vi "Filter.vi"(8 "error in (no error)":errorcluster, 10 "Input":sgl[][](array[numeric]), 11 "Std. Deviation in":refnum<class "Std. Deviation.lvclass">) -> (0 "error out":errorcluster, 2 "Output":sgl[][](array[numeric]), 3 "Std. Deviation out":refnum<class "Std. Deviation.lvclass">)   [LabVIEW 2015, in "Std. Deviation.lvclass"]
uses:
  Std. Deviation.lvclass
  Std. Deviation.lvclass/Std. Deviation.ctl
  Filter.lvclass
  <vilib>/Analysis/NI_AALBase.lvlib
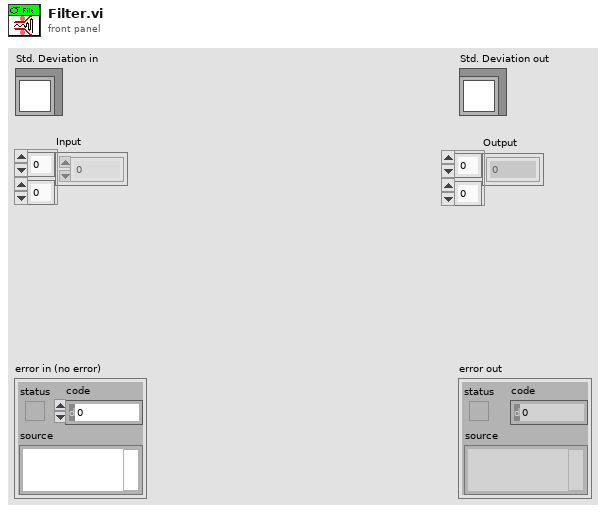
[diagram p1: front panel]
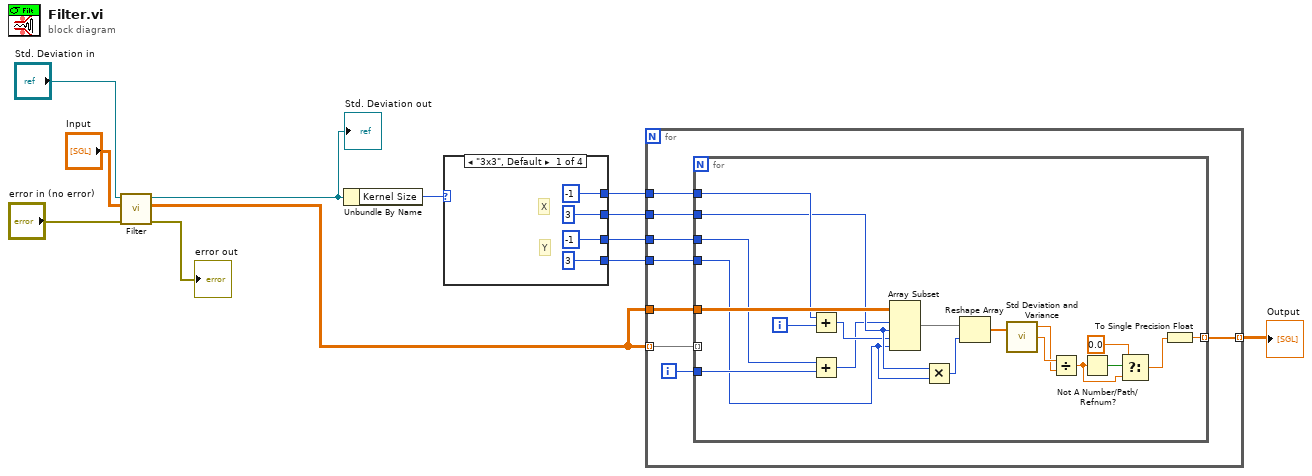
[diagram p0: block diagram]
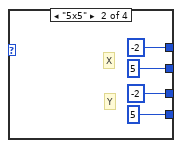
[diagram p2: hidden frame]
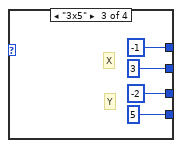
[diagram p3: hidden frame]
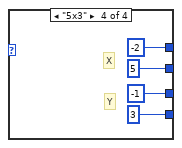
[diagram p4: hidden frame]
diagram:
  n1 = call-parent "Filter.vi"("error in (no error)"="error in (no error)", "Input"="Input", "Filter in"="Std. Deviation in") -> ("error out"=→"error out":errorcluster, "Output"=w7:sgl[][], "Filter out"=w1:refnum<class "Std. Deviation.lvclass">)  [unwired: 6 in]
  "Std. Deviation out" <- w1
  n2 = Unbundle By Name(w1) -> ("Kernel Size"=w8:enum16{"3x3", "5x5", "3x5", "5x3"})
  n3 = case shown="\"3x3\", Default" w8 {
    tunnel: [-1 -2 -1 -2] -> w6
    tunnel: [3 5 3 5] -> w5
    tunnel: [-1 -2 -2 -1] -> w4
    tunnel: [3 5 5 3] -> w3
    frame "3x3", Default {
      # "Y"
      # "X"
    }
    frame "5x5" {
      # "Y"
      # "X"
    }
    frame "3x5" {
      # "Y"
      # "X"
    }
    frame "5x3" {
      # "Y"
      # "X"
    }
  }
  n4 = for {
    tunnel: w7 -> [w36] mode=indexing
    tunnel: w7 -> [w35]
    tunnel: w6 -> [w34]
    tunnel: w5 -> [w33]
    tunnel: w4 -> [w32]
    tunnel: w3 -> [w30]
    tunnel: [w29] -> w2 mode=indexing
    i -> [w31]
    n5 = for {
      tunnel: w36 -> [_] mode=indexing
      tunnel: w35 -> [w55]
      tunnel: w34 -> [w53]
      tunnel: w33 -> [w49]
      tunnel: w32 -> [w52]
      tunnel: w31 -> [w51]
      tunnel: w30 -> [w48]
      tunnel: [w45] -> w29 mode=indexing
      i -> [w54]
      n6 = Add(x=w53, y=w54) -> (x+y=w38:i32)
      n7 = Add(x=w52, y=w51) -> (x+y=w37:i32)
      n8 = Array Subset(array=w55, index (row)=w37, length (row)=w49, index (col)=w38, length (col)=w48) -> (w50:sgl[][])
      n9 = Multiply(x=w49, y=w48) -> (x*y=w47:i32)
      n10 = Reshape Array(w50, w47) -> (w46:sgl[])
      n11 = call <vilib>:"Std Deviation and Variance.vi"("X"=w46) -> ("mean"=w43:dbl, "standard deviation"=w44:dbl)  [unwired: 1 in, 1 out]
      n12 = Divide(x=w44, y=w43) -> (x/y=w40:dbl)
      n13 = Not A Number/Path/Refnum?(number/path/refnum=w40) -> (NaN/Path/Refnum?=w42:bool)
      n14 = Select(t=0.0, s=w42, f=w40) -> (s? t:f=w39:dbl)
      n15 = To Single Precision Float(number=w39) -> (single precision float=w45:sgl)
    }
  }
  "Output" <- w2
